vi "AuMT8852B Path Offset Table Entry.vi"(5 "Offset (0 dBm)":dbl format="%.2f", 6 "Frequency units (Channel)":enum16{"Channel", "MHz"}(ring), 7 "Set/Get (Set)":enum16{"Set", "Get"}(ring), 8 "error in (no error)":errorcluster, 9 "Frequency (Channel 0)":i32, 10 "Table (1)":i32=1, 11 "VISA session":refnum<visa-resource-name>) -> (0 "error out":errorcluster, 2 "error code":i32, 3 "VISA session out":refnum<visa-resource-name>, 4 "Offset out":dbl format="%.2f")   [LabVIEW 2017]
doc: "Anritsu MT8852B Bluetooth Tester\n\nSpecifies an offset for a particular frequency or channel in the selected path offset table.\n\nINPUTS\nSet/Get - whether the value is being sent to or retrieved from the instrument.\nTable - path offset table (1-10) to use.\nFrequency - frequency at which the offset will be applied.\nFrequency units - whether the frequency is expressed as a channel or a frequency in MHz.\nOffset - path offset to apply at the given frequency or channel.\n\nOUTPUTS\nOffset out - path offset currently being used at the given frequency or channel."
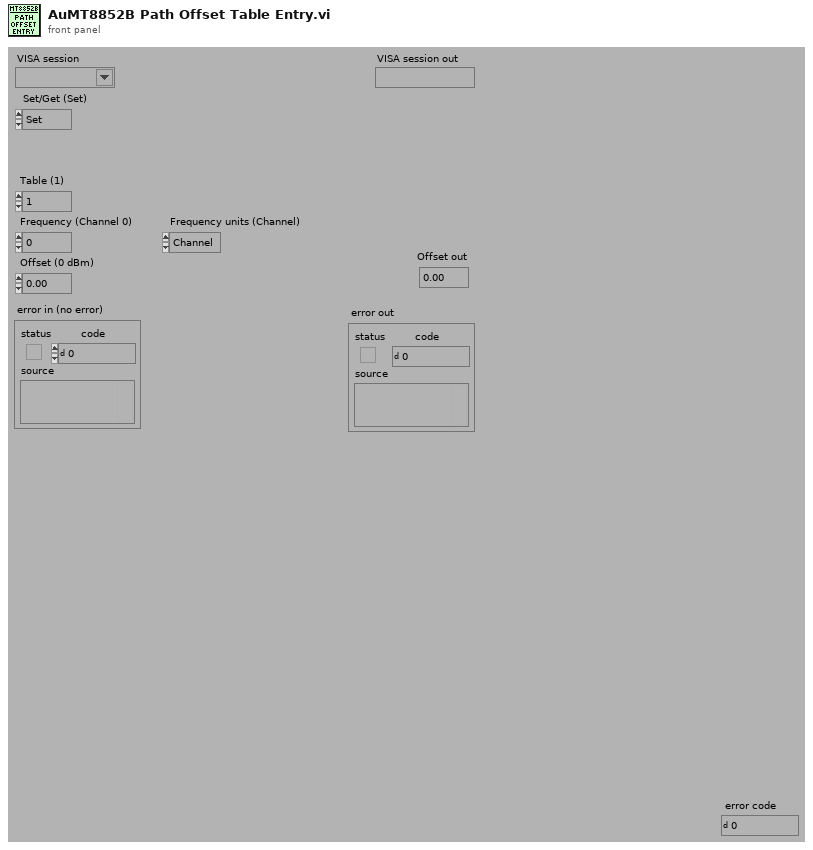
[diagram p1: front panel]
types:
  T1 = enum16{"Simulate", "Range check", "Cache", "Query instrument status"}
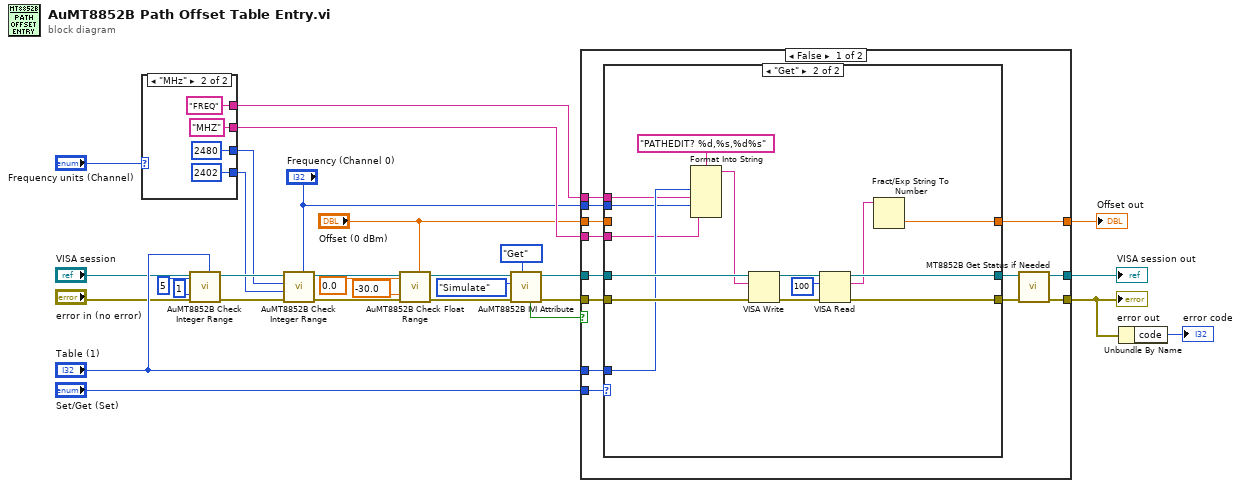
[diagram p0: block diagram]
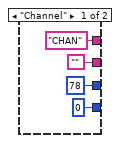
[diagram p2: hidden frame]
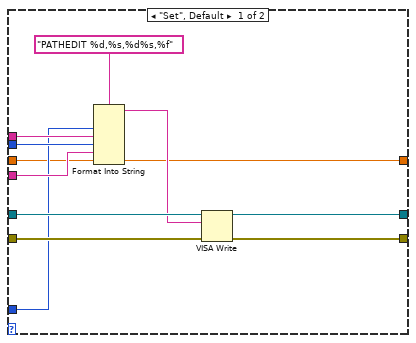
[diagram p3: hidden frame]
diagram:
  n1 = case shown="\"MHz\"" "Frequency units (Channel)" {
    tunnel: [0 2402] -> w16
    tunnel: [78 2480] -> w15
    tunnel: ["" "MHZ"] -> w5
    tunnel: ["CHAN" "FREQ"] -> w2
    frame "Channel" {
    }
    frame "MHz" {
    }
  }
  n2 = call <instrlib>:"AuMT8852B Check Integer Range.vi"("Value (0)"="Table (1)", "error in (no error)"="error in (no error)", "Lower limit (-1)"=1, "Upper limit (1)"=5, "VISA session"="VISA session") -> ("error out"=w19:errorcluster, "VISA session out"=w18:refnum<visa-resource-name>)  [unwired: 5 in]
  n3 = call <instrlib>:"AuMT8852B Check Integer Range.vi"("Value (0)"="Frequency (Channel 0)", "error in (no error)"=w19, "Lower limit (-1)"=w16, "Upper limit (1)"=w15, "VISA session"=w18) -> ("error out"=w14:errorcluster, "VISA session out"=w13:refnum<visa-resource-name>)  [unwired: 5 in]
  n4 = call <instrlib>:"AuMT8852B Check Float Range.vi"("Value (0)"="Offset (0 dBm)", "error in (no error)"=w14, "Lower limit (-1)"=-30.0, "Upper limit (1)"=0.0, "VISA session"=w13) -> ("error out"=w11:errorcluster, "VISA session out"=w12:refnum<visa-resource-name>)  [unwired: 5 in]
  n5 = call <instrlib>:"AuMT8852B IVI Attribute.vi"("Set/Get (Set)"=enum16{"Set", "Get"}."Get", "error in (no error)"=w11, "Flag (Simulate)"=T1."Simulate", "VISA session"=w12) -> ("error out"=w28:errorcluster, "VISA session out"=w29:refnum<visa-resource-name>, "Value out"=w25:bool)  [unwired: 5 in]
  n6 = case shown="False" w25 {
    tunnel: [w44 w80] -> w30
    tunnel: [w45 w79] -> w23
    tunnel: w29 -> [w51 w80]
    tunnel: w28 -> [w50 w79]
    tunnel: "Set/Get (Set)" -> [w49 _]
    tunnel: "Table (1)" -> [w48 _]
    tunnel: w5 -> [w43 _]
    tunnel: "Frequency (Channel 0)" -> [w42 _]
    tunnel: "Offset (0 dBm)" -> [w41 w78]
    tunnel: w2 -> [w40 _]
    tunnel: [w39 w78] -> w1
    frame False {
      n7 = case shown="\"Get\"" w49 {
        tunnel: w51 -> [w60 w77]
        tunnel: w50 -> [w61 w76]
        tunnel: [w57 w69] -> w47
        tunnel: w48 -> [w53 w67]
        tunnel: [w58 w70] -> w46
        tunnel: w43 -> [w55 w64]
        tunnel: w42 -> [w56 w65]
        tunnel: w41 -> [w52 _]
        tunnel: w40 -> [w54 w66]
        tunnel: [w52 w63] -> w39
        frame "Set", Default {
          n8 = Format Into String(format string="PATHEDIT %d,%s,%d%s,%f" ("Command ()"), w53, w54, w56, w55, w52) -> (resulting string=w59:string)  [unwired: 2 in, 1 out]
          n9 = VISA Write(VISA resource name=w60, write buffer=w59, error in (no error)=w61) -> (VISA resource name out=w58:refnum<visa-resource-name>, error out=w57:errorcluster)  [unwired: 1 out]
        }
        frame "Get" {
          n10 = Format Into String(format string="PATHEDIT? %d,%s,%d%s" ("Format String"), w67, w66, w65, w64) -> (resulting string=w71:string)  [unwired: 2 in, 1 out]
          n11 = VISA Write(VISA resource name=w77, write buffer=w71, error in (no error)=w76) -> (VISA resource name out=w74:refnum<visa-resource-name>, error out=w75:errorcluster)  [unwired: 1 out]
          n12 = VISA Read(VISA resource name=w74, byte count=u32 100 ("byte count (0)"), error in (no error)=w75) -> (VISA resource name out=w70:refnum<visa-resource-name>, read buffer=w68:string, error out=w69:errorcluster)  [unwired: 1 out]
          n13 = Fract/Exp String To Number(string=w68) -> (number=w63:dbl)  [unwired: 3 in, 1 out]
        }
      }
      n14 = call <instrlib>:"MT8852B Get Status if Needed.vi"("error in (no error)"=w47, "VISA session"=w46) -> ("error out"=w45:errorcluster, "VISA session out"=w44:refnum<visa-resource-name>)  [unwired: 8 in]
    }
    frame True {
      (unwired) "" ("Response")
    }
  }
  "error out" <- w23
  "VISA session out" <- w30
  "Offset out" <- w1
  n15 = Unbundle By Name(w23) -> ("code"=→"error code":i32)
